vi "Actor Core.vi"(8 "error in":errorcluster, 11 "UIA_ChildTestMaster in":refnum<class "UIA_ChildTestMaster.lvclass">) -> (0 "error out":errorcluster, 3 "Actor out":refnum<class "Actor.lvclass">)   [LabVIEW 2020, in "UIA_ChildTestMaster.lvlib" / "UIA_ChildTestMaster.lvclass"]
doc: "(<B>Filename</B>: Actor Framework.lvlib:Actor.lvclass:Actor Core.vi)\n\nReceives messages to the actor, reacts to them, and initiates any error handling that may shut the actor down.\n\nDescendant classes may override this VI to append parallel tasks for the actor to complete while it handles messages. Overrides use the Call Parent Method node."
uses:
  UIA_ChildTestMaster.lvclass
  D:/Projets/STEP AT/UI Actor/UI_Actor/UI_Actor/UI_Actor.lvclass
  support/Actor Framework.lvlibp/1abvi3w/vi.lib/ActorFramework/Actor/Actor.lvclass
  UIA_ChildTest/UIA_ChildTest/UIA_ChildTest.lvclass
  UI_Actor/UI_Actor Messages/UI_ShowIn_FreeWindow Msg/UI_ShowIn_FreeWindow Msg.lvclass/UI_ShowIn_FreeWindow Msg.ctl
  support/Actor Framework.lvlibp/1abvi3w/vi.lib/ActorFramework/Message Enqueuer/Enqueue.vi
  UI_Actor/UI_Actor Messages/UI_ShowIn_FreeWindow Msg/UI_ShowIn_FreeWindow Msg.lvclass
  UI_Actor/UI_Actor/UI_Actor.lvclass
panel:
  out "S2.indic":dbl caption="Ctl1"
  out "S1.Ctl1":dbl caption="Ctl1"
  # "UI ACTOR CHILDTEST Master\n\nINTERFACE DE TEST"
  # "Je gère un CHILDTEST Nested ^^"
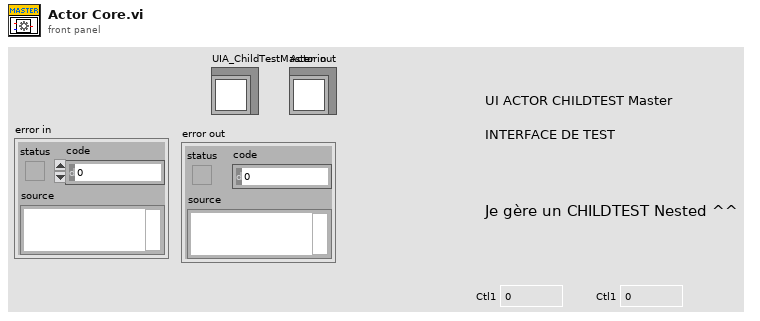
[diagram p1: front panel]
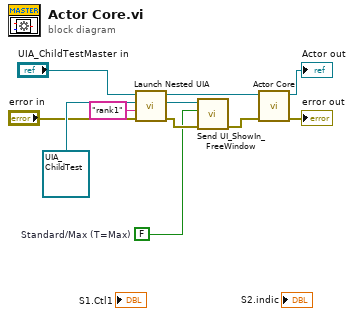
[diagram p0: block diagram]
diagram:
  w1 = FALSE  # Standard/Max (T=Max)
  n1 = call "Launch Nested UIA.vi"("error in (no error)"="error in", "Name"="rank1", "UI_Actor"=refnum<class "UIA_ChildTest.lvclass"> refnum ("UIA_ChildTest.lvlib:UIA_ChildTest.lvclass"), "Caller UIA in"="UIA_ChildTestMaster in") -> ("error out"=w4:errorcluster, "Nested Actor's Enqueuer"=w5:refnum<class "Message Enqueuer.lvclass">, "Caller UIA out"=w8:refnum<class "UIA_ChildTestMaster.lvclass">)  [unwired: 5 in]
  n2 = call "Send UI_ShowIn_FreeWindow.vi"("error in (no error)"=w4, "Standard/Max (T=Max)"=w1, "Message Enqueuer"=w5) -> ("error out"=w3:errorcluster)  [unwired: 7 in, 1 out]
  n3 = call-parent "Actor Core.vi"("error in"=w3, "UI_Actor in"=w8) -> ("error out"=→"error out":errorcluster, "Actor out"=→"Actor out":refnum<class "Actor.lvclass">)  [unwired: 8 in]
